vi "CRYStep Setup Replace Open VI.vi"(4 "Step Name":string, 6 "StepNo.":i32, 8 "sData":string, 9 "sOption":string, 10 "VI Path":path, 11 "Category":string) -> (0 "pVIRefStepSubVI":refnum<vi>, 2 "pVIRef":refnum<vi>)   [LabVIEW 2013]
uses:
  CRYStepSetup/CRYStepSetup Global.vi
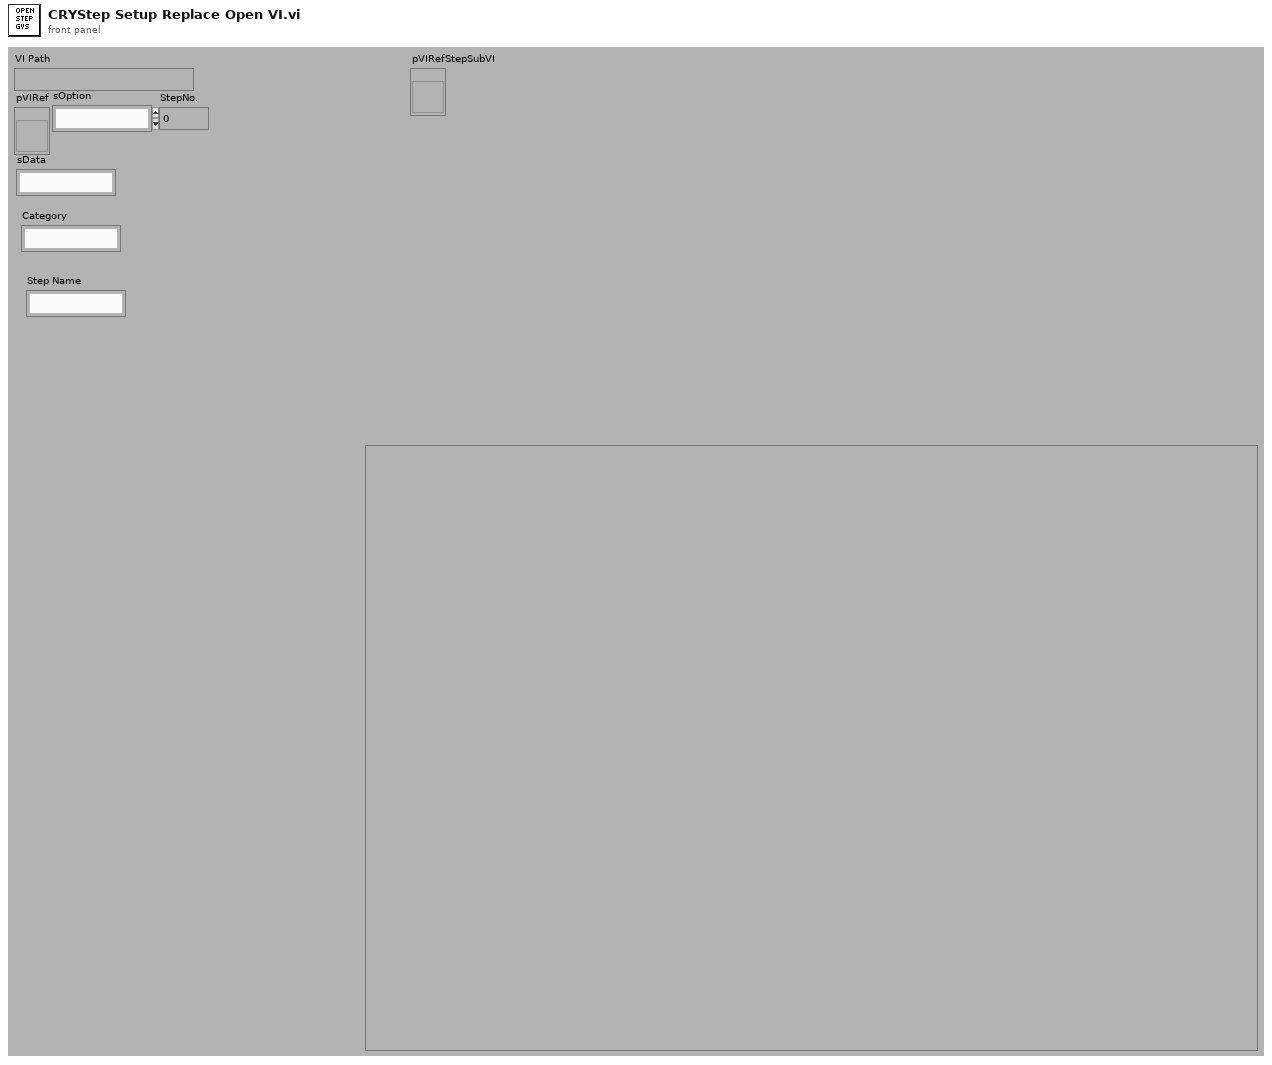
[diagram p1: front panel]
types:
  T1 = cluster{"nID":i32, "sTiltle":string, "pVI":refnum<vi>, "pSP":refnum<vi>, "pTab":refnum<vi>, "pSPT":refnum<vi>, "nWinType":i32, "sIcon":string}
  T2 = cluster{"nID":i32, "sName":string, "sType":string, "sProperty":string, "sTemplet":string, "sDocking":string, "pVIRef":refnum<vi>, "pSPRef":refnum<vi>, "pRefTemplet":refnum<vi>, "pRefSplitter":refnum<vi>[], "nPosSplitter":i32[], "pRefSP":refnum<vi>[], "nSPID":i32[], "sSPDock":string[], "nIDFrame":i32[], "nIDPanel":i32[], "nActiveFrame":i32, "nCountFrame":i32, "cFrame":cluster{"nID":i32, "sName":string, "sType":string, "sTitle":string, "sIcon":string, "pVIRef":refnum<vi>, "pSPRef":refnum<vi>, "cWiin":cluster{"sName":string, "sType":string, "pVIRef":refnum<vi>, "sData":string}, "cTab":cluster{"sTitle":string, "sIcon":string, "pSpliter":refnum<vi>, "nAvtivePage":i32, "nIDPage":i32[], "nIDFrame":i32[]}, "sData":string}[], "sData":string, "sSplitterName":string[]}
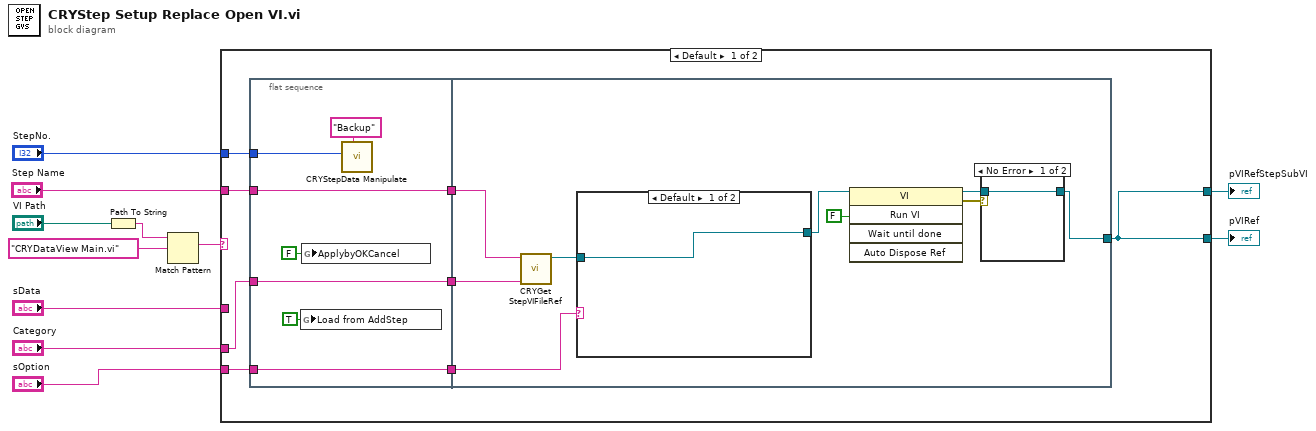
[diagram p0: block diagram]
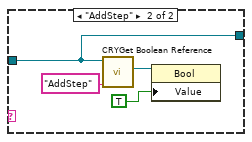
[diagram p2: hidden frame]
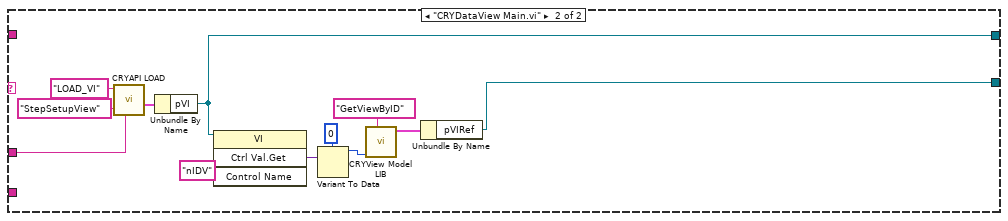
[diagram p4: hidden frame]
diagram:
  n1 = Path To String(path="VI Path") -> (string=w3:string)
  n2 = Match Pattern(string=w3, regular expression="CRYDataView Main.vi" ("string")) -> (match substring=w9:string)  [unwired: 1 in, 3 out]
  n3 = case shown="Default" w9 {
    tunnel: [w19 w43] -> w10
    tunnel: "sData" -> [_ w53]
    tunnel: [w19 w44] -> w7
    tunnel: "Category" -> [w18 _]
    tunnel: "sOption" -> [w17 _]
    tunnel: "StepNo." -> [w14 _]
    tunnel: "Step Name" -> [w13 _]
    frame Default {
      n4 = flat-sequence {
        tunnel: w17 -> [w25]
        tunnel: w18 -> [w26]
        tunnel: [w26] -> w16
        tunnel: [w25] -> w15
        tunnel: w14 -> [w23]
        tunnel: w13 -> [w21]
        tunnel: [w21] -> w12
        tunnel: [w32] -> w19
        tunnel: w16 -> [w31]
        tunnel: w15 -> [w29]
        tunnel: w12 -> [w27]
        frame #0 {
          n5 = global write "CRYStepSetup Global.vi" "Load from AddStep"(TRUE ("Load from AddStep")) -> ()
          n6 = global write "CRYStepSetup Global.vi" "ApplybyOKCancel"(FALSE ("ApplybyOKCancel")) -> ()
          n7 = call "CRYStepData Manipulate.vi"("sAction"="Backup", "StepNo."=w23) -> ()  [unwired: 10 in]
        }
        frame #1 {
          n8 = call "CRYGet StepVIFileRef.vi"("Category"=w31, "Step Name"=w27) -> ("Step Edit VI ref"=w30:refnum<vi>)  [unwired: 6 in, 2 out]
          n9 = case shown="Default" w29 {
            tunnel: w30 -> [w36 w37]
            tunnel: [w36 w37] -> w28
            frame Default {
            }
            frame "AddStep" {
              n10 = call "CRYGet Boolean Reference.vi"("Label Name"="AddStep", "VI Refnum"=w37) -> ("Boolean Ref"=w38:refnum<vi>)  [unwired: 9 out]
              n11 = property class="Bool"(reference=w38, "Value"=TRUE) -> ()  [unwired: 1 in, 2 out]
            }
          }
          n12 = invoke class="VI" method="Run VI"(reference=w28, "Wait until done"=FALSE ("Wait Until Done")) -> (reference out=w34:refnum<vi>, error out=w33:errorcluster)  [unwired: 3 in, 3 out]
          n13 = case shown="No Error" w33 {
            tunnel: [w41 w42] -> w32
            tunnel: w34 -> [w41 w42]
            frame No Error {
            }
            frame Error {
            }
          }
        }
      }
    }
    frame "CRYDataView Main.vi" {
      n14 = call "CRYAPI LOAD.vi"("sOption"=w53, "sData"="StepSetupView", "sAction"="LOAD_VI") -> ("tWindow_Out"=w51:T1)  [unwired: 5 in, 3 out]
      n15 = Unbundle By Name(w51) -> ("pVI"=w44:refnum<vi>)
      n16 = invoke class="VI" method="Ctrl Val.Get"(reference=w44, "Control Name"="nIDV") -> ("Get Control Value Variant"=w47:variant)  [unwired: 2 in, 3 out]
      n17 = Variant To Data(type=0, Variant=w47) -> (data=w50:i32)  [unwired: 1 in, 1 out]
      n18 = call "CRYView Model LIB.vi"("sAction"="GetViewByID", "nData"=w50) -> ("cView_Out"=w45:T2)  [unwired: 7 in, 2 out]
      n19 = Unbundle By Name(w45) -> ("pVIRef"=w43:refnum<vi>)
    }
  }
  "pVIRef" <- w10
  "pVIRefStepSubVI" <- w7
